vi "PPS_DRIVE_GET_GYRO.vi"() -> (3 "Gyro Heading Radians":dbl)   [LabVIEW 2019]
uses:
  PPS_DRIVE_GLOBALS.vi
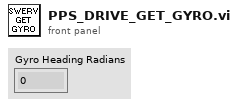
[diagram p1: front panel]
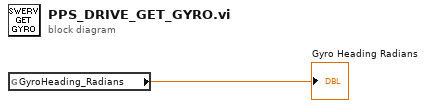
[diagram p0: block diagram]
diagram:
  n1 = global read "PPS_DRIVE_GLOBALS.vi" "GyroHeading_Radians"() -> (→"Gyro Heading Radians":dbl)
